vi "set_settings_cluster.vi"(8 "error in (no error)":errorcluster, 10 "settings cluster in":variant, 11 "ImagingModeDL100901FlexTrajectory in":refnum<class "ImagingModeDL100901FlexTrajectory.lvclass">) -> (0 "error out":errorcluster, 3 "ImagingModeDL100901FlexTrajectory out":refnum<class "ImagingModeDL100901FlexTrajectory.lvclass">)   [LabVIEW 2010, in "ImagingModeDL100901FlexTrajectory.lvclass"]
uses:
  ImagingModeDL100901FlexTrajectory.lvclass
  ImagingModeDL100901FlexTrajectory.lvclass/ImagingModeDL100901FlexTrajectory.ctl
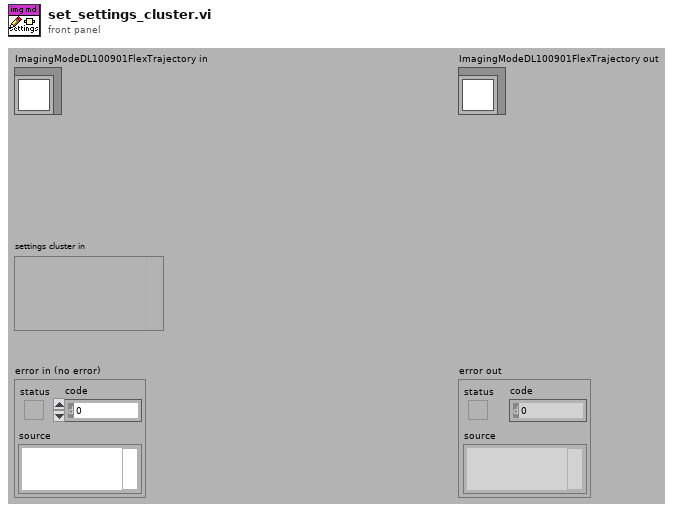
[diagram p1: front panel]
types:
  T1 = typedef "ImagingModeDL100901FlexTrajectory.lvclass/settings_cluster.ctl" = cluster{"ScanRepetitions":i32, "LinesPerFrame":i32, "ScanRate":dbl[unit]}
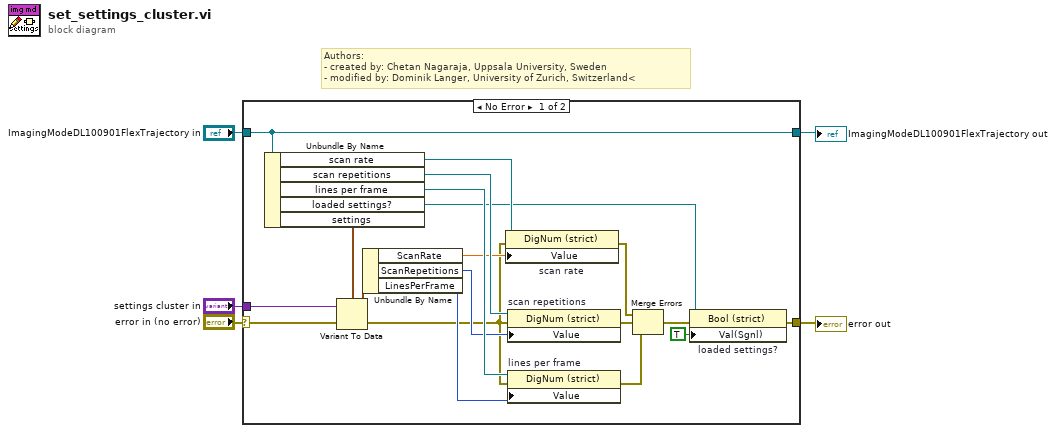
[diagram p0: block diagram]
diagram:
  # "Authors: \n- created by: Chetan Nagaraja, Uppsala University, Sweden\n- modified by: Dominik Langer, University of Zurich, Switzerland<"
  n1 = case shown="No Error" "error in (no error)" {
    selector: "error in (no error)" -> [w15 w26]
    tunnel: "ImagingModeDL100901FlexTrajectory in" -> [w13 w25]
    tunnel: [w9 w26] -> w3
    tunnel: [w13 w25] -> w2
    tunnel: "settings cluster in" -> [w14 _]
    frame No Error {
      n2 = Unbundle By Name(w13) -> ("scan rate"=w19:refnum<vi>, "scan repetitions"=w23:refnum<vi>, "lines per frame"=w22:refnum<vi>, "loaded settings?"=w8:refnum<vi>, "settings"=w12:T1)
      n3 = Variant To Data(error in=w15, Variant=w14, type=w12) -> (error out=w10:errorcluster, data=w24:T1)
      n4 = Unbundle By Name(w24) -> ("ScanRate"=w18:dbl[unit], "ScanRepetitions"=w21:i32, "LinesPerFrame"=w20:i32)
      n5 = property on="scan rate" class="DigNum (strict)"(reference=w19, error in=w10, "Value"=w18) -> (error out=w11:errorcluster)  [unwired: 1 out]
      n6 = property on="scan repetitions" class="DigNum (strict)"(reference=w23, error in=w10, "Value"=w21) -> (error out=w17:errorcluster)  [unwired: 1 out]
      n7 = property on="lines per frame" class="DigNum (strict)"(reference=w22, error in=w10, "Value"=w20) -> (error out=w16:errorcluster)  [unwired: 1 out]
      n8 = Merge Errors(w11, w17, w16) -> (w7:errorcluster)
      n9 = property on="loaded settings?" class="Bool (strict)"(reference=w8, error in=w7, "Val(Sgnl)"=TRUE ("Value (Signaling)")) -> (error out=w9:errorcluster)  [unwired: 1 out]
    }
    frame Error {
    }
  }
  "error out" <- w3
  "ImagingModeDL100901FlexTrajectory out" <- w2
